vi "FTW-Publisher-Destroy.vi"(0 "FTW-Publisher In":refnum<class "FTW-Publisher.lvclass">, 11 "error in":errorcluster) -> (15 "error out":errorcluster)   [LabVIEW 2013, in "FTW-Publisher.lvclass"]
uses:
  FTW-Publisher.lvclass
  <vilib>/event_ctls.llb/usereventprio.ctl
  FTW-Publisher.lvclass/FTW-Publisher.ctl
  Endpoint/FTW-Endpoint.lvclass
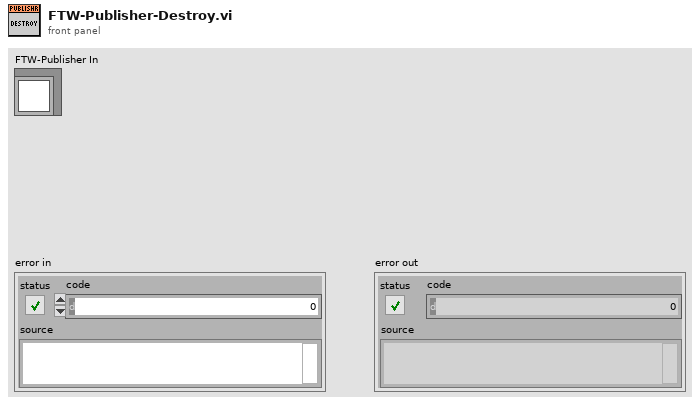
[diagram p1: front panel]
types:
  T1 = typedef "usereventprio.ctl" = enum32{"high priority", "normal priority"}
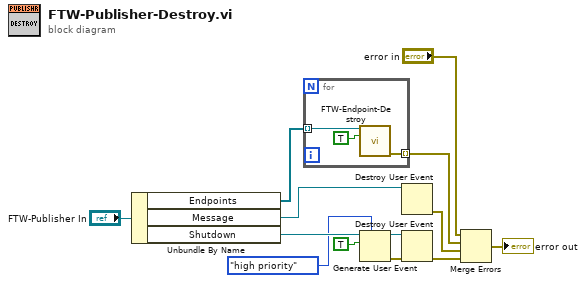
[diagram p0: block diagram]
diagram:
  n1 = Unbundle By Name("FTW-Publisher In") -> ("Endpoints"=w9:refnum<class "FTW-Endpoint.lvclass">[], "Message"=w10:refnum<user-event>, "Shutdown"=w6:refnum<user-event>)
  n2 = for {
    tunnel: w9 -> [w16] mode=indexing
    tunnel: [w15] -> w8 mode=indexing
    n3 = call-dynamic "FTW-Endpoint-Destroy.vi"("FTW Endpoint"=w16, "Force Destroy"=TRUE) -> ("error out"=w15:errorcluster)  [unwired: 13 in]
  }
  n4 = Generate User Event(priority (normal)=usereventprio."high priority", user event=w6, event data cluster=TRUE ("event data")) -> (user event out=w4:refnum<user-event>, error out=w3:errorcluster)  [unwired: 1 in]
  n5 = Destroy User Event(user event=w10) -> (error out=w7:errorcluster)  [unwired: 1 in]
  n6 = Destroy User Event(user event=w4, error in=w3) -> (error out=w5:errorcluster)
  n7 = Merge Errors("error in", w8, w7, w5) -> (→"error out":errorcluster)
